vi "Get real location.vi"(2 "error in":errorcluster, 3 "Image":T1) -> (0 "error out":errorcluster, 1 "Matches":T2[](array[typedef]) {"Correlation Score" format="%.2f"; "Target Template Curve Score" format="%.2f"; "Template Target Curve Score" format="%.2f"; "Bounding Box"."y" format="%.2f"; "Bounding Box"."x" format="%.2f"; "Position"."y" format="%.2f"; "Position"."x" format="%.2f"; "Score" format="%.2f"; "Scale" format="%.2f"; "Angle" format="%.2f"; "Occlusion %" format="%.2f"})   [LabVIEW 2011]
uses:
  <vilib>/vision/Pattern Matching.llb/IMAQ GM Match Report.ctl
  <vilib>/vision/Image Controls.llb/IMAQ Image.ctl
  <vilib>/vision/Pattern Matching.llb/IMAQ Curve Parameters.ctl
  <vilib>/vision/Pattern Matching.llb/IMAQ Match Range Setting.ctl
panel:
  out "Templete Image":T1(plugin-control)
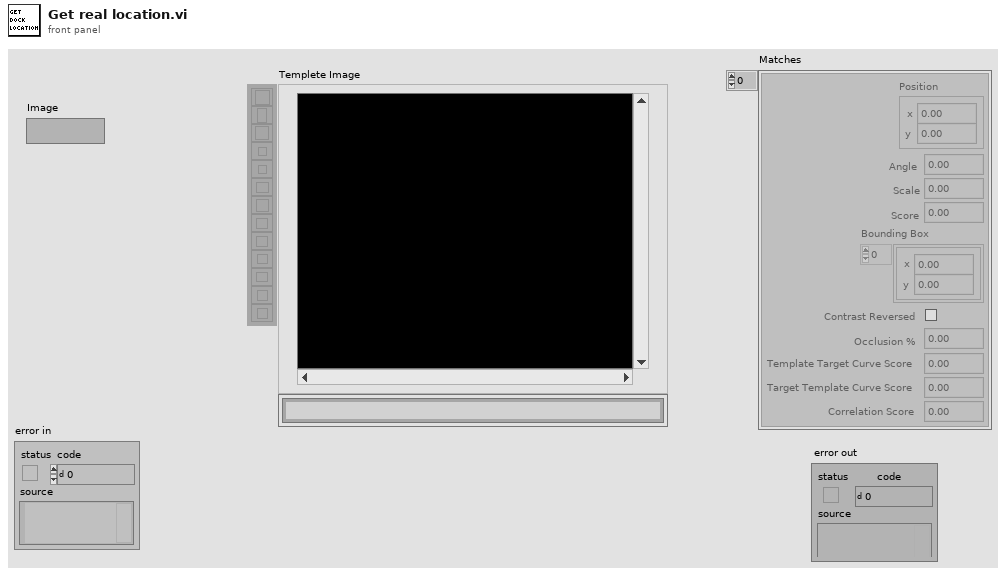
[diagram p1: front panel]
types:
  T1 = typedef "IMAQ Image.ctl" = refnum<image>
  T2 = typedef "IMAQ GM Match Report.ctl" = cluster{"Position":cluster{"x":sgl, "y":sgl}, "Angle":sgl, "Scale":sgl, "Score":sgl, "Bounding Box":cluster{"x":sgl, "y":sgl}[], "Contrast Reversed":bool, "Occlusion %":sgl, "Template Target Curve Score":sgl, "Target Template Curve Score":sgl, "Correlation Score":sgl}
  T3 = typedef "IMAQ Curve Parameters.ctl" = cluster{"Extraction Mode":u32, "Edge Threshold":i32, "Edge Filter Size":u32, "Min Length":i32, "Row Search Step Size":i32, "Col Search Step Size":i32, "Max Endpoint Gap":i32, "Closed":bool, "Subpixel":bool}
  T4 = typedef "IMAQ Match Range Setting.ctl" = cluster{"Match Constraints":u32, "Min":dbl, "Max":dbl}
  T5 = cluster{"Curve Parameters":T3, "Match Mode":cluster{"Rotation":bool, "Scale":bool, "Occlusion":bool, "Reserved":bool, "Reserved":bool, "Reserved":bool}, "Range Settings":T4[], "Number of Matches":i32, "Minimum Match Score":sgl, "SubPixel Accuracy":bool, "Adv. Geometric Match Options 2":cluster{"Setup Data Item":u16, "Item Value":dbl}[]}
  T6 = cluster{"Global Rectangle":i32[], "Contours":cluster{"ID":enum32{"External", "Internal"}, "Type":u32, "Coordinates":i32[]}[]}
  T7 = typedef "Image Type" = u32
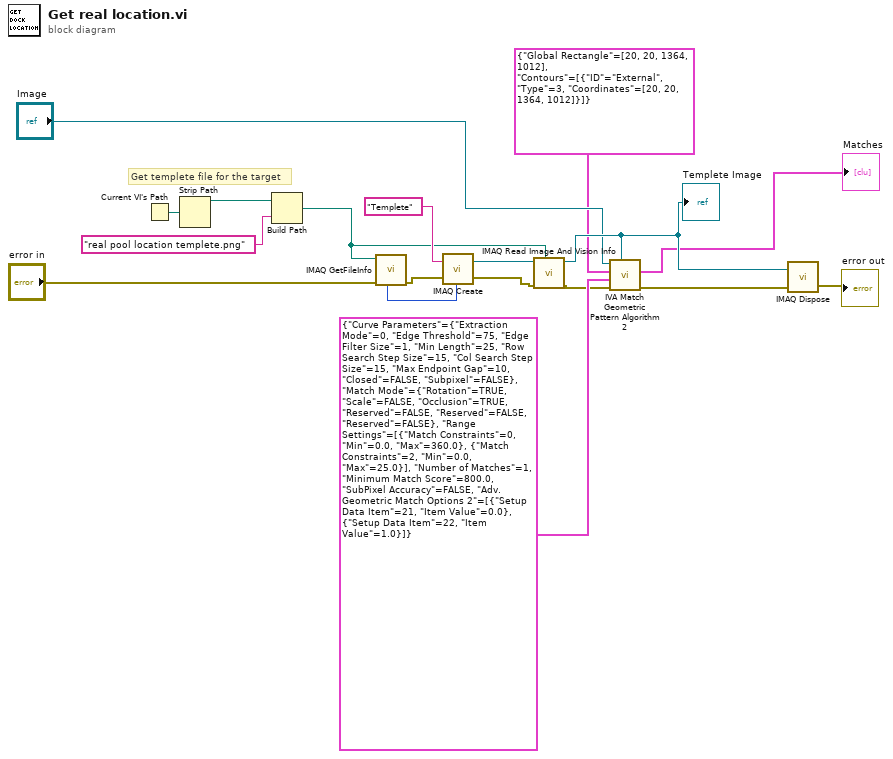
[diagram p0: block diagram]
diagram:
  # "Get templete file for the target"
  n1 = Current VI's Path() -> (path=w16:path)
  n2 = Strip Path(path=w16) -> (stripped path=w15:path)  [unwired: 1 out]
  n3 = Build Path(base path=w15, name or relative path="real pool location templete.png") -> (appended path=w11:path)
  n4 = call "IMAQ GetFileInfo"("error in (no error)"="error in", "File Path"=w11) -> ("error out"=w14:errorcluster, "Image Type"=w13:T7)  [unwired: 3 in, 5 out]
  n5 = call "IMAQ Create"("Image Name"="Templete", "Image Type"=w13, "error in (no error)"=w14) -> ("New Image"=w9:T1, "error out"=w10:errorcluster)  [unwired: 1 in, 1 out]
  n6 = call "IMAQ Read Image And Vision Info"("File Path"=w11, "error in (no error)"=w10, "Image"=w9) -> ("error out"=w3:errorcluster, "Image Out"=w7:T1)  [unwired: 1 in, 6 out]
  "Templete Image" <- w7
  n7 = call <vilib>:"IVA Match Geometric Pattern Algorithm 2.vi"("Template"=w7, "error in (no error)"=w3, "Settings"=T5 {"Curve Parameters"={"Extraction Mode"=0, "Edge Threshold"=75, "Edge Filter Size"=1, "Min Length"=25, "Row Search Step Size"=15, "Col Search Step Size"=15, "Max Endpoint Gap"=10, "Closed"=FALSE, "Subpixel"=FALSE}, "Match Mode"={"Rotation"=TRUE, "Scale"=FALSE, "Occlusion"=TRUE, "Reserved"=FALSE, "Reserved"=FALSE, "Reserved"=FALSE}, "Range Settings"=[{"Match Constraints"=0, "Min"=0.0, "Max"=360.0}, {"Match Constraints"=2, "Min"=0.0, "Max"=25.0}], "Number of Matches"=1, "Minimum Match Score"=800.0, "SubPixel Accuracy"=FALSE, "Adv. Geometric Match Options 2"=[{"Setup Data Item"=21, "Item Value"=0.0}, {"Setup Data Item"=22, "Item Value"=1.0}]} ("Settings (Geometric Matching 1)"), "ROI Descriptor"=T6 {"Global Rectangle"=[20, 20, 1364, 1012], "Contours"=[{"ID"=enum."External", "Type"=3, "Coordinates"=[20, 20, 1364, 1012]}]} ("ROI Descriptor (Geometric Matching 1)"), "Image"="Image") -> ("error out"=w1:errorcluster, "Matches"=→"Matches":T2[])  [unwired: 1 in, 4 out]
  n8 = call "IMAQ Dispose"("Image"=w7, "error in (no error)"=w1) -> ("error out"=→"error out":errorcluster)  [unwired: 4 in]
